vi "Read SSL Context.vi"(8 "error in (no error)":errorcluster, 11 "SSL Context in":refnum<class "SSL Context.lvclass">) -> (0 "error out":errorcluster, 2 "SSL_Lib.lvlib:SSL-Context.lvclass":refnum<class "SSL-Context.lvclass">, 3 "SSL Context out":refnum<class "SSL Context.lvclass">)   [LabVIEW 2013, in "OpenSSL Socket.lvlib" / "SSL Context.lvclass"]
uses:
  SSL Context.lvclass
  SSL_Lib/SSL-Context/SSL-Context.lvclass
  SSL Context.lvclass/SSL Context.ctl
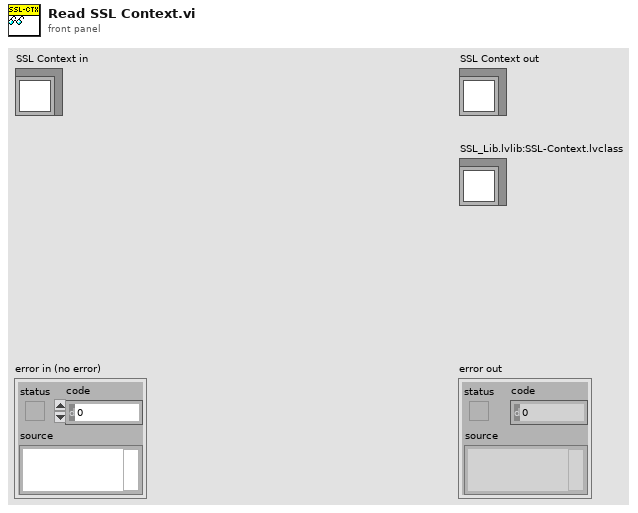
[diagram p1: front panel]
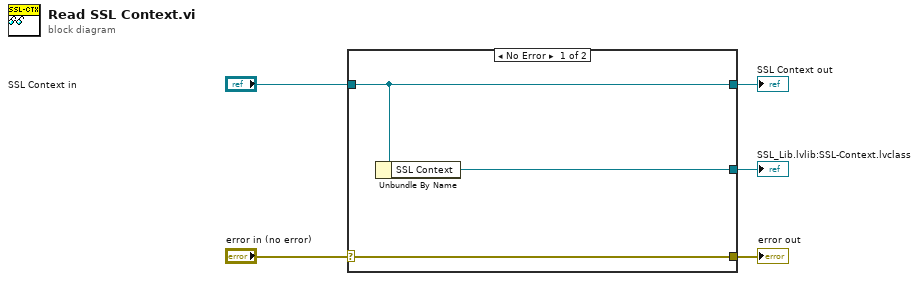
[diagram p0: block diagram]
diagram:
  n1 = case shown="No Error" "error in (no error)" {
    selector: "error in (no error)" -> [w8 w9]
    tunnel: [w8 w9] -> w4
    tunnel: [w7 w10] -> w2
    tunnel: "SSL Context in" -> [w7 w10]
    tunnel: [w6 _] -> w1
    frame No Error {
      n2 = Unbundle By Name(w7) -> ("SSL Context"=w6:refnum<class "SSL-Context.lvclass">)
    }
    frame Error {
    }
  }
  "error out" <- w4
  "SSL Context out" <- w2
  "SSL_Lib.lvlib:SSL-Context.lvclass" <- w1
